vi "GyroTurn.vi"() -> ()   [LabVIEW 2016, in "LEGO-PMR.lvrbt"]
uses:
  LEGO-PMR.lvrbt
  <vilib>/NXT/Block Support/NXT_InputPort.ctl
  <vilib>/NXT/Block Support/NXT_OutputPort.ctl
  <vilib>/NXT/Dual Mode Library/Sensors/EV3_Gyro_Reset.vi
  <vilib>/NXT/Dual Mode Library/Sensors/EV3_Gyro_Angle.vi
  <vilib>/NXT/NXTIO Xnodes/NXTIONodeSubVIs/NXTMoveMotors.vi
  <vilib>/NXT/Dual Mode Library/Waits/Wait_Num.vi
  <vilib>/NXT/NXTIO Xnodes/AddressXNode/NXTIOAddress.xnode
  <vilib>/NXT/NXTIO Xnodes/NXTIOXNode/NXTIO.xnode
  <vilib>/NXT/Subs/LVHSConnector.ctl
  <vilib>/NXT/LegoClasses/BrickReference/BrickReference.lvclass
panel:
  in  "Speed":dbl
  in  "Angle (negative version) dumbass":dbl
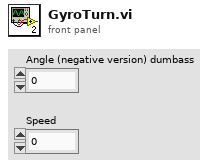
[diagram p1: front panel]
types:
  T1 = typedef "NXT_InputPort.ctl" = u32
  T2 = typedef "LVHSConnector.ctl" = refnum<class "BrickReference.lvclass">
  T3 = typedef "NXT_OutputPort.ctl" = u8
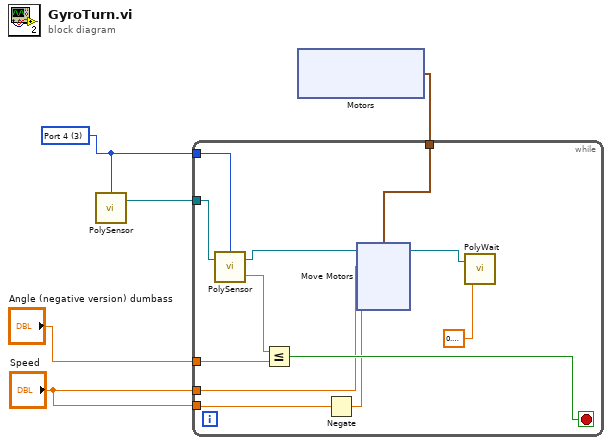
[diagram p0: block diagram]
diagram:
  w1 = T1 3 items=["Port 1", "Port 2", "Port 3", "Port 4"] ("Port (Port 1)")
  n1 = call-poly <vilib>:"PolySensor.vi"("Port (Port 1)"=w1) -> ("NXT/EV3"=w3:T2)  [unwired: 3 in]
  n2 = xnode "Motors"() -> ("Motor"=w4:cluster{"Port":T3, "Port":T3})
  n3 = while {
    tunnel: "Angle (negative version) dumbass" -> [w16]
    tunnel: w4 -> [w14]
    tunnel: w3 -> [w12]
    tunnel: "Speed" -> [w11]
    tunnel: "Speed" -> [w7]
    tunnel: w1 -> [w10]
    stop <- w15 stop-if-true
    n4 = call-poly <vilib>:"PolySensor.vi"("NXT/EV3"=w12, "Port (Port 1)"=w10) -> ("Degrees"=w17:sgl, "NXT/EV3"=w13:T2)  [unwired: 1 in]
    n5 = Less Or Equal?(x=w17, y=w16) -> (x <= y?=w15:bool)
    n6 = Negate(x=w7) -> (-x=w6:dbl)
    n7 = xnode "Move Motors"("Power/Speed 2"=w6, "Power/Speed 1"=w11, "Motors"=w14, "NXT/EV3"=w13) -> ("NXT/EV3"=w8:T2)
    n8 = call-poly <vilib>:"PolyWait.vi"("Time (1 sec)"=0.10000000000000002, "NXT/EV3"=w8) -> ()  [unwired: 2 in, 1 out]
  }
